vi "GenerateTargetArrayForRange.vi"(1 "LeftHand":bool, 2 "Min Range":dbl, 3 "Max Range":dbl, 4 "Starting Position":dbl) -> (0 "Target Array":dbl[](array[numeric]))   [LabVIEW 2015]
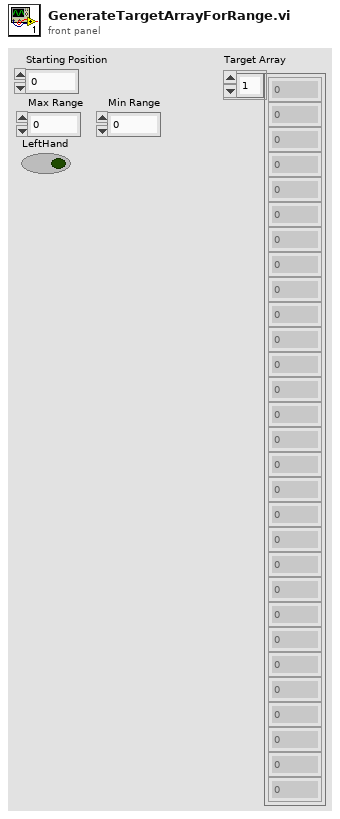
[diagram p1: front panel]
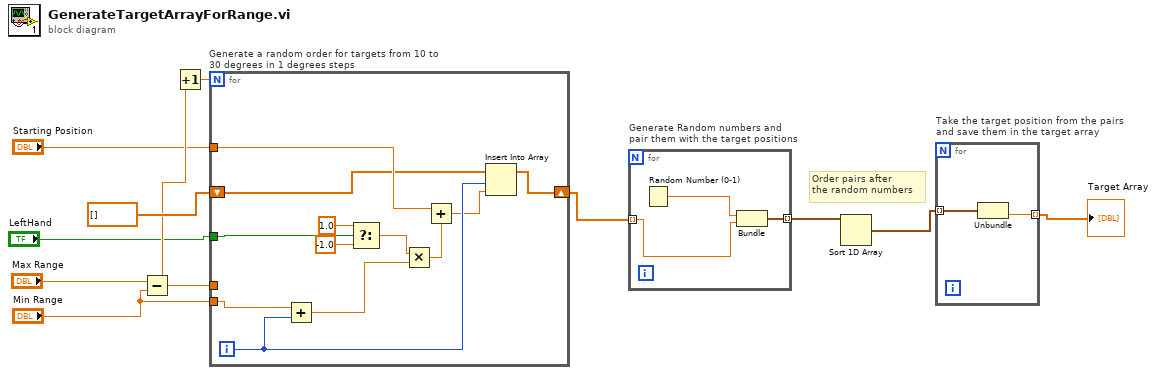
[diagram p0: block diagram]
diagram:
  # "Order pairs after\nthe random numbers"
  n1 = Subtract(x="Max Range", y="Min Range") -> (x-y=w7:dbl)
  n2 = Increment(x=w7) -> (x+1=w6:dbl)
  n3 = for "Generate a random order for targets from 10 to 30 degrees in 1 degrees steps" {
    N: w6 -> [_]
    tunnel: w7 -> [_]
    tunnel: "Starting Position" -> [w19]
    tunnel: "LeftHand" -> [w23]
    tunnel: "Min Range" -> [w14]
    shift-right: [w16] -> w8
    shift-left: dbl[] [] -> [w17]
    i -> [w15]
    n4 = Add(x=w14, y=w15) -> (x+y=w13:dbl)
    n5 = Select(t=1.0, s=w23, f=-1.0) -> (s? t:f=w20:dbl)
    n6 = Multiply(x=w20, y=w13) -> (x*y=w18:dbl)
    n7 = Add(x=w19, y=w18) -> (x+y=w12:dbl)
    n8 = Insert Into Array(array=w17, index=w15, new element=w12) -> (w16:dbl[])
  }
  n9 = for "Generate Random numbers and \npair them with the target positions" {
    tunnel: w8 -> [w25] mode=indexing
    tunnel: [w24] -> w10 mode=indexing
    n10 = Random Number (0-1)() -> (number: 0 to 1=w26:dbl)
    n11 = Bundle("number: 0 to 1"=w26, w25) -> (w24:cluster{"number: 0 to 1":dbl, dbl})  [unwired: 1 in]
  }
  n12 = Sort 1D Array(array=w10) -> (sorted array=w9:cluster{"number: 0 to 1":dbl, dbl}[])
  n13 = for "Take the target position from the pairs\nand save them in the target array" {
    tunnel: w9 -> [w28] mode=indexing
    tunnel: [w27] -> w5 mode=indexing
    n14 = Unbundle(w28) -> (w27:dbl)  [unwired: 1 out]
  }
  "Target Array" <- w5
